vi "Folder Hierarchy Verifier.vi"() -> ()   [LabVIEW 2023]
doc: "Displays a window to view the expected folder hierarchy on disk and and compare it to the actual folder hierarchy."
uses:
  CTLs/Folder Verifier State Data.ctl
  <userlib>/_MGI/Application Control/MGI Gray if/MGI Gray if False.vi
  SubVIs/FaKI State Machine/FaKI State Machine.lvlib
panel:
  in  "Flat Constructors?":bool
  in  "Project Hierarchy":string(tree)
  in  "Analyze Project":bool
  in  "Exit":bool
  in  "Project File":path
  # "A non-container project item will be red if expected path does not match actual path. A container project item will be red if none of the containing expected paths match actual paths, purple if some match and some don't match, and dark red if non-container items directly below it do not share a common directory"
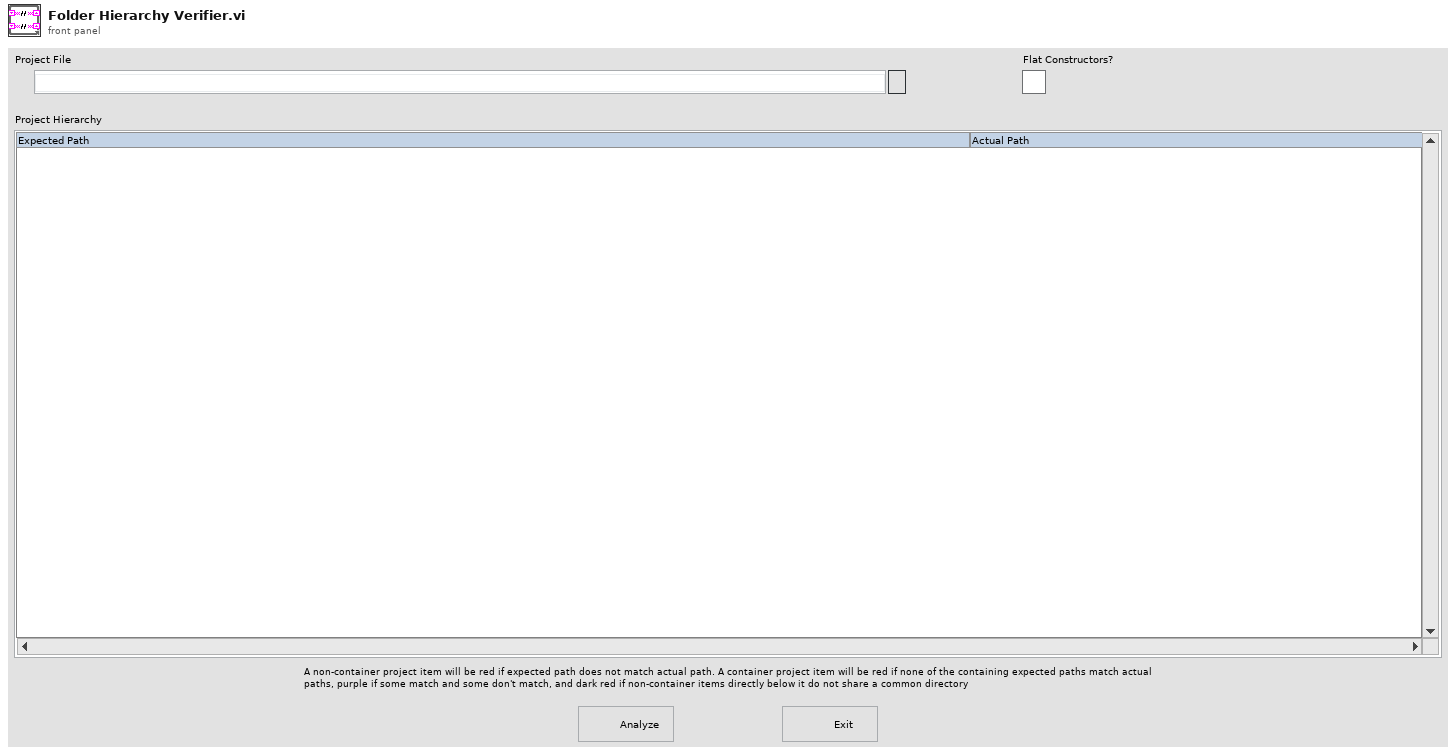
[diagram p1: front panel]
types:
  T1 = typedef "Folder Verifier State Data.ctl" = cluster{"Core":cluster{"Current VI Reference":refnum<vi>, "Close Panel on Exit?":bool}, "Tree Refnum":refnum<vi>, "Project":path, "Expected Paths":path[], "Actual Paths":path[]}
  T2 = enum32{"Invalid", "Standard", "Closed", "Hidden", "Minimized", "Maximized"}
  T3 = enum32{"invalid app kind", "Development System", "Run Time System", "Student Edition", "Embedded LabVIEW", "Evaluation", "Custom"}
  T4 = enum8{"Enabled", "Disabled", "Disabled and Grayed Out"}
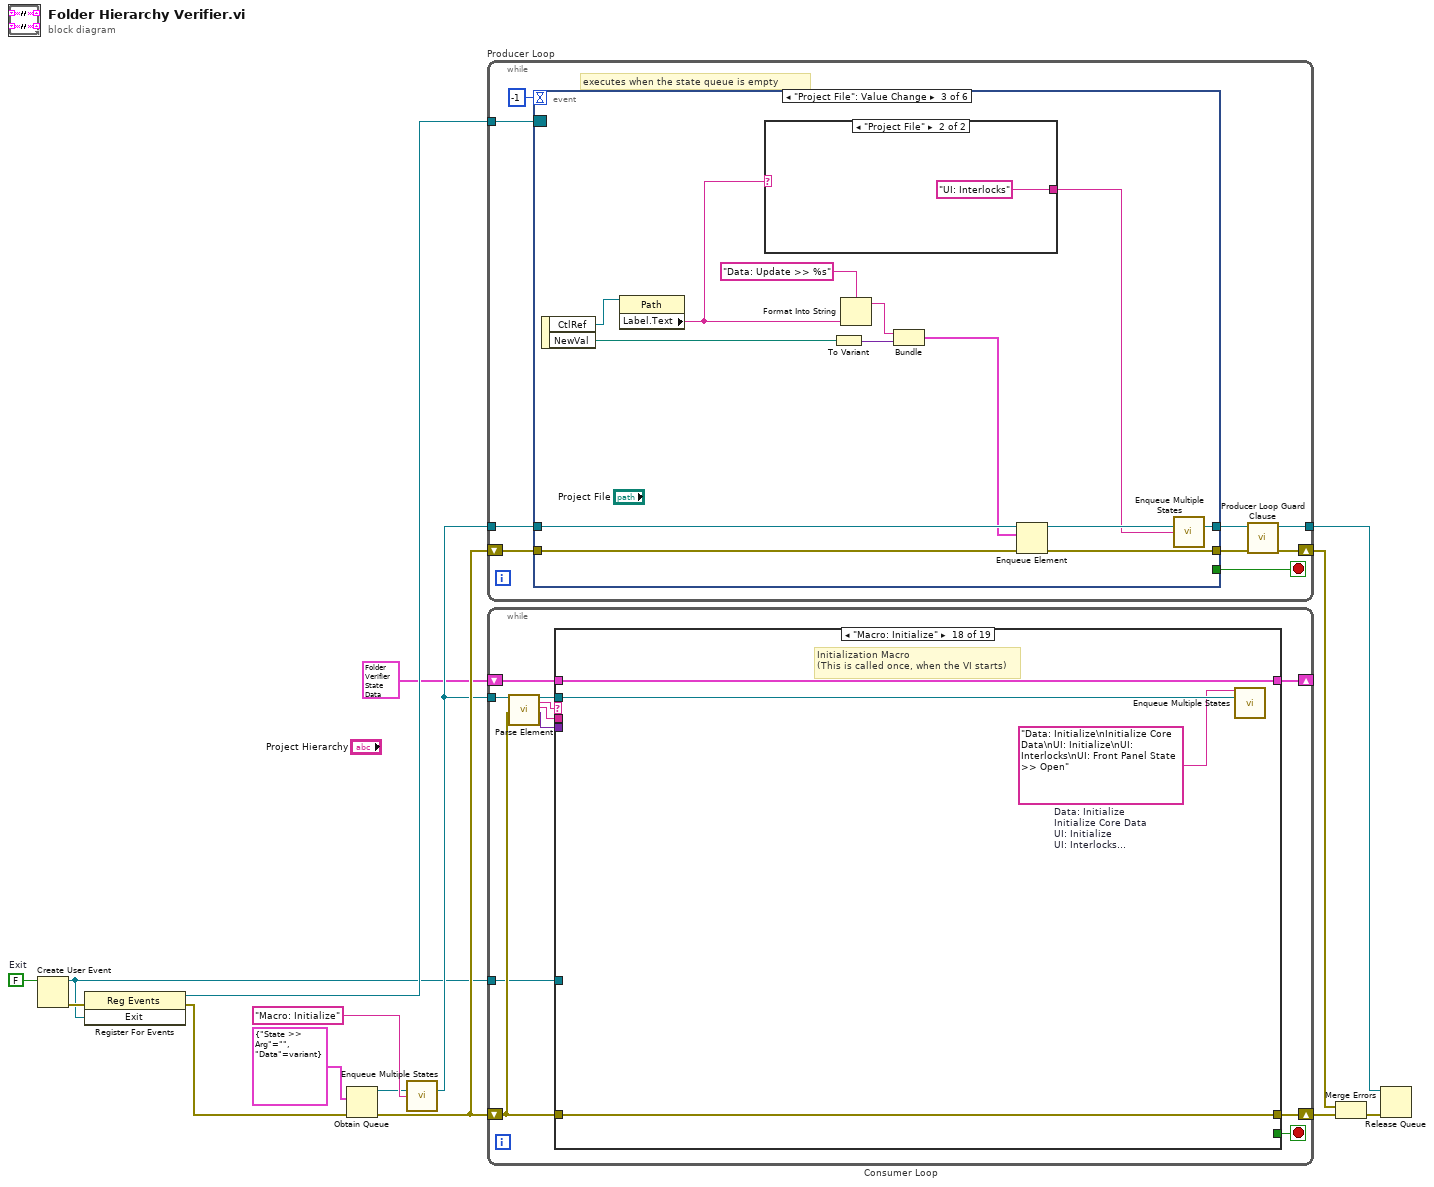
[diagram p0: block diagram]
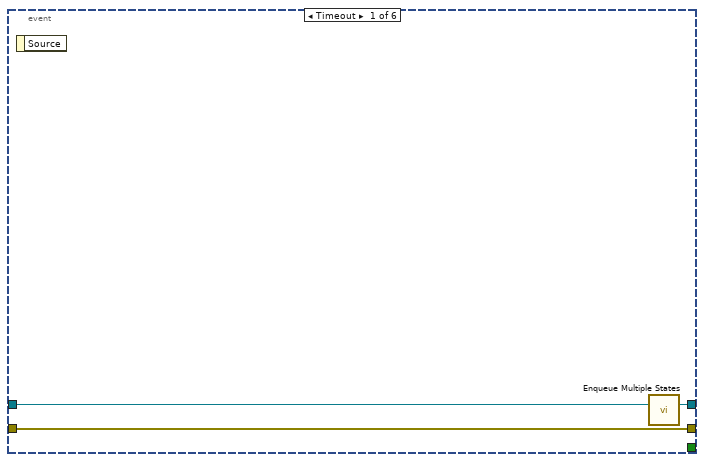
[diagram p2: hidden frame]
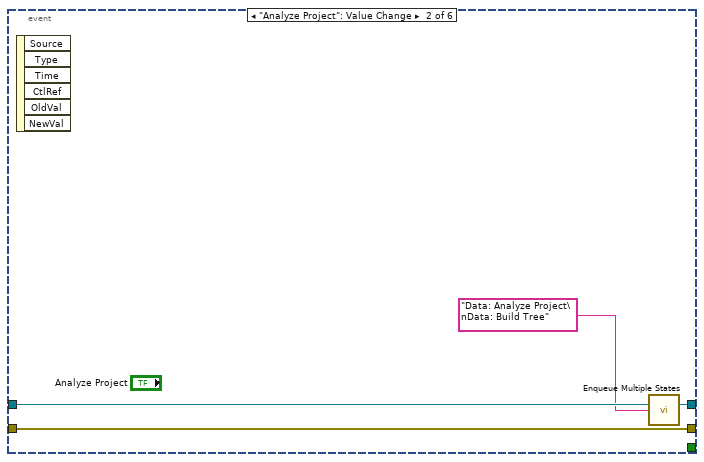
[diagram p3: hidden frame]
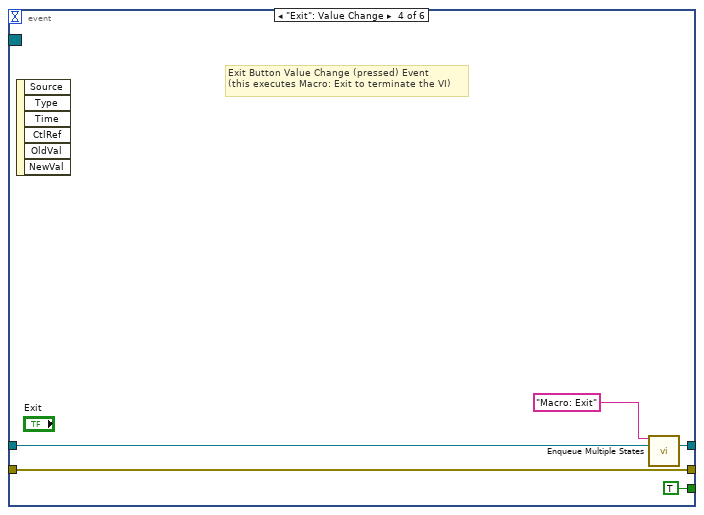
[diagram p5: hidden frame]
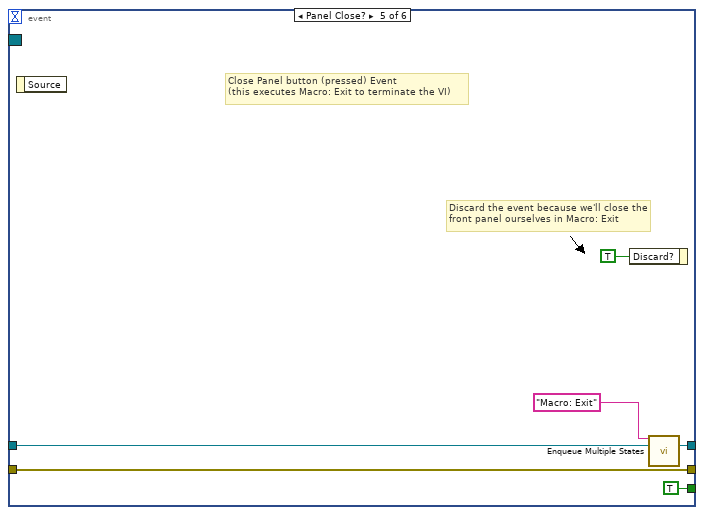
[diagram p6: hidden frame]
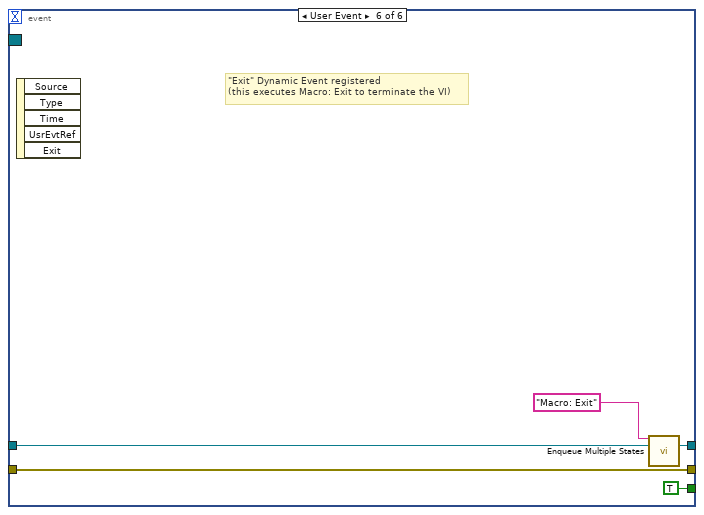
[diagram p7: hidden frame]
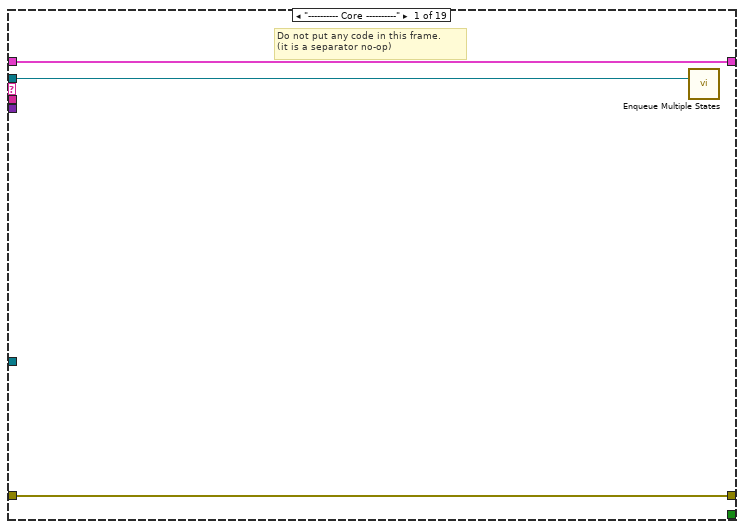
[diagram p8: hidden frame]
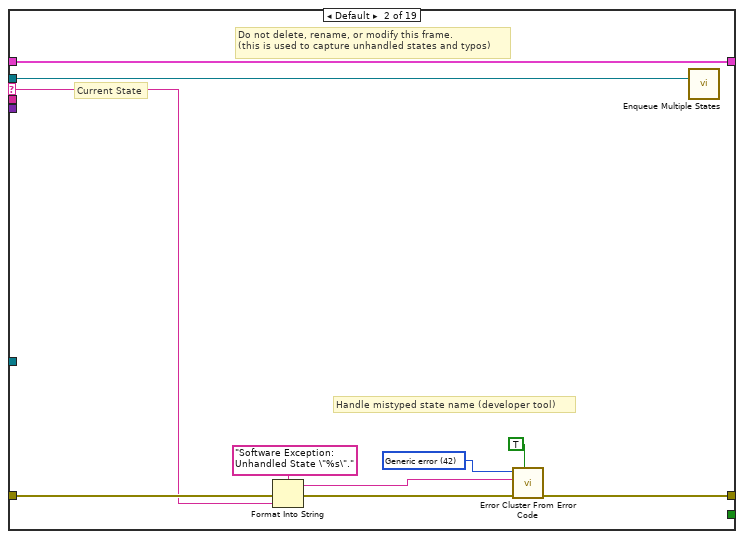
[diagram p9: hidden frame]
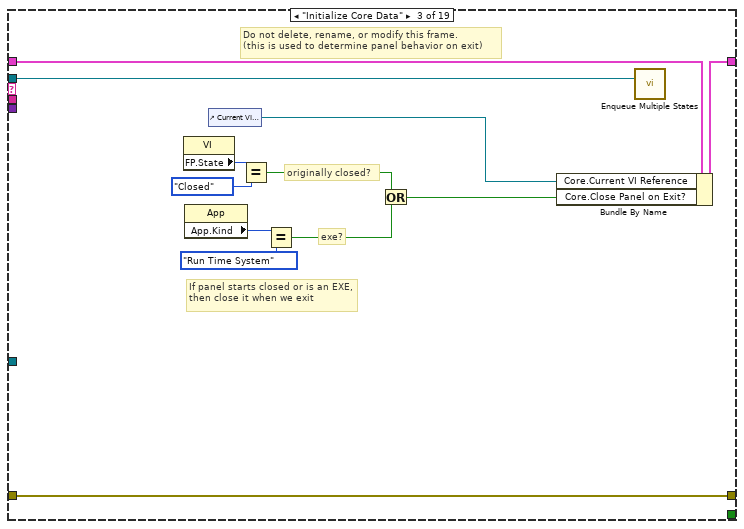
[diagram p10: hidden frame]
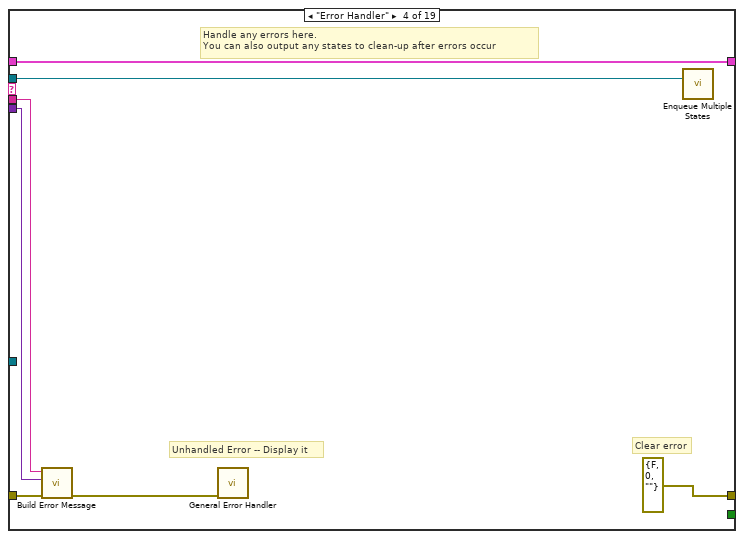
[diagram p11: hidden frame]
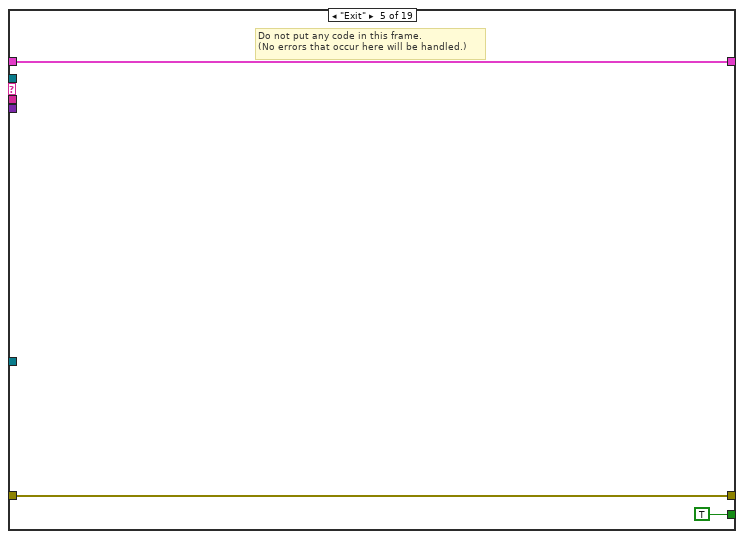
[diagram p12: hidden frame]
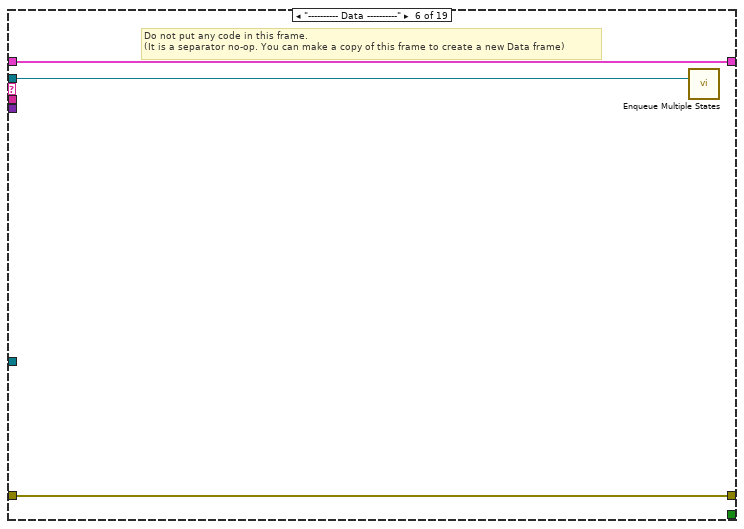
[diagram p13: hidden frame]
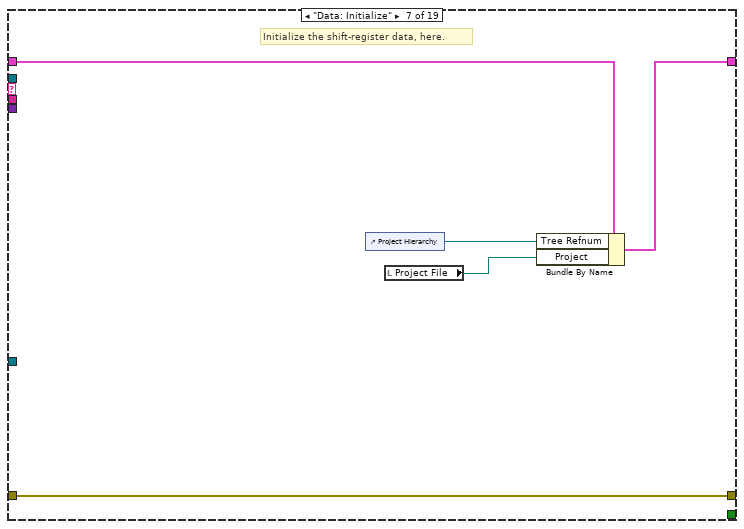
[diagram p14: hidden frame]
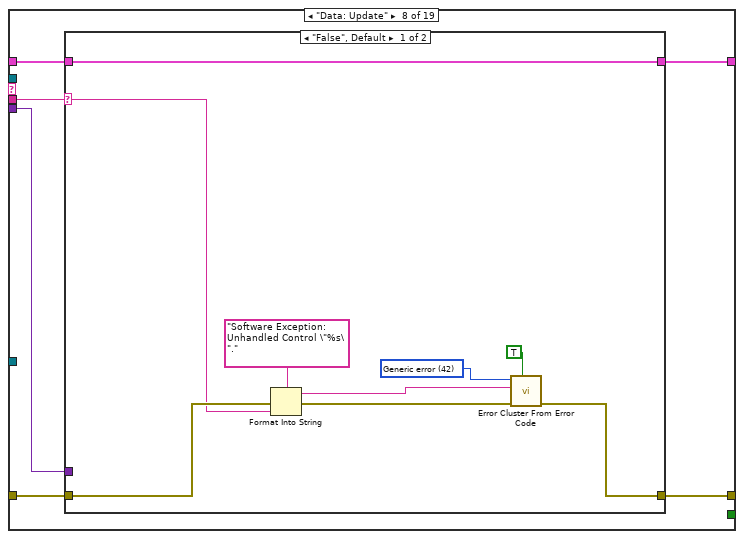
[diagram p15: hidden frame]
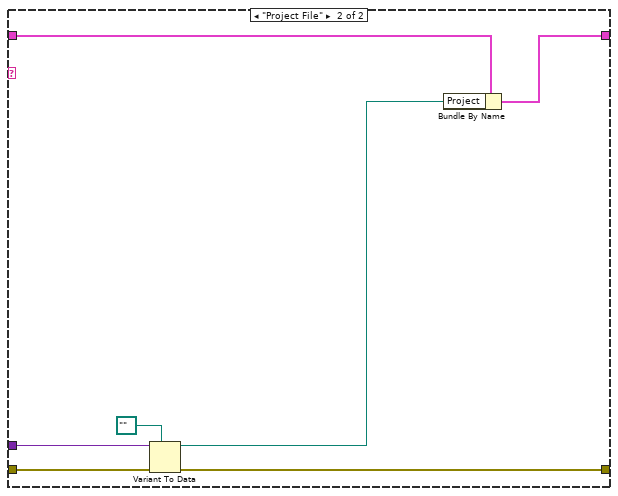
[diagram p16: hidden frame]
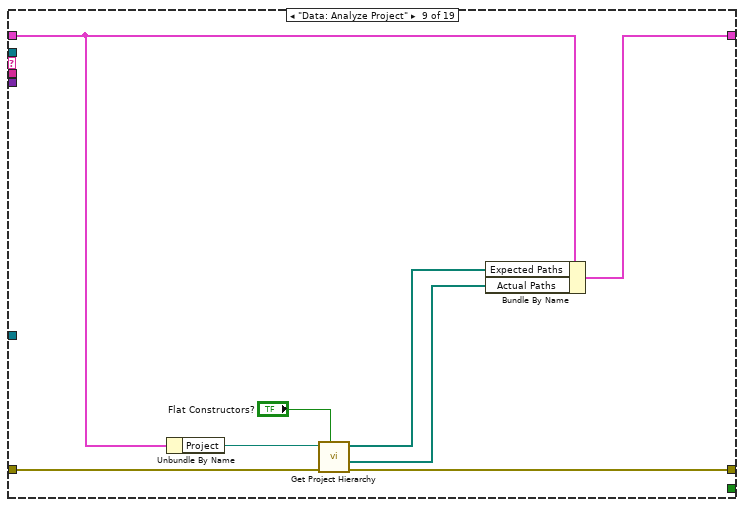
[diagram p17: hidden frame]
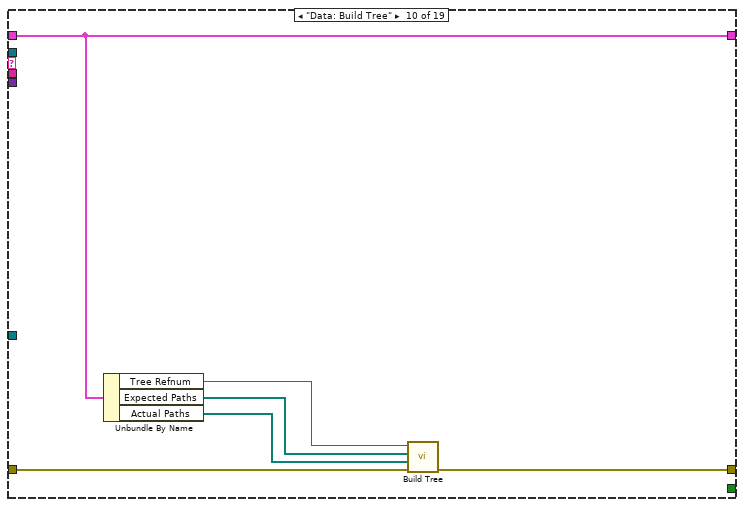
[diagram p18: hidden frame]
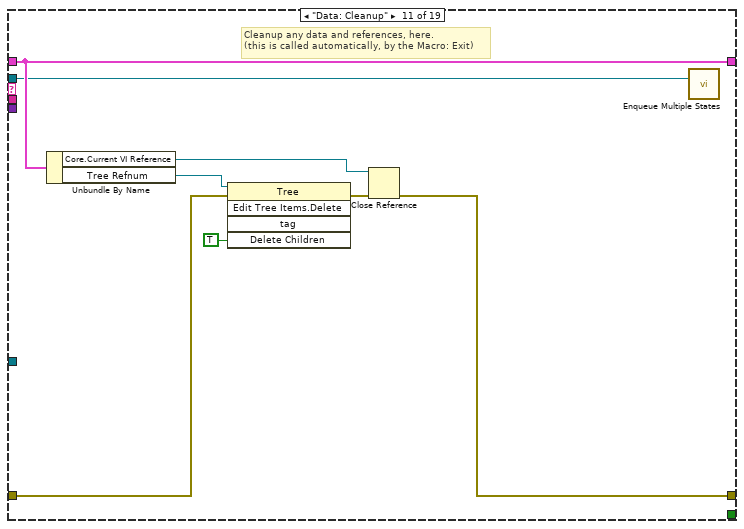
[diagram p19: hidden frame]
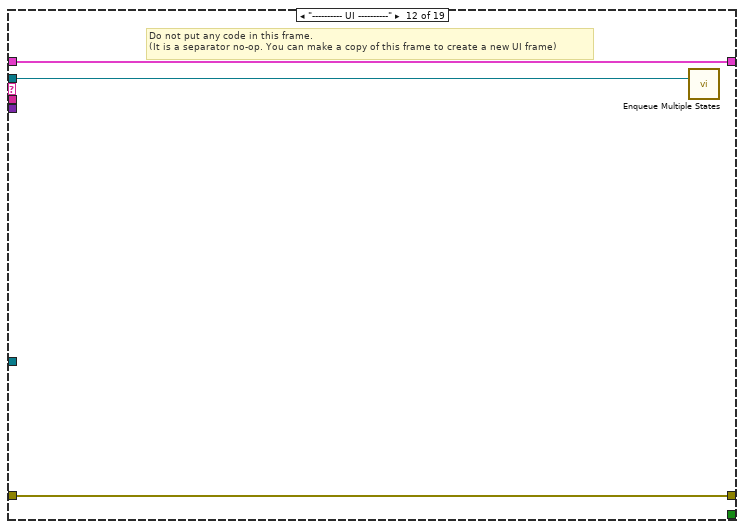
[diagram p20: hidden frame]
diagram:
  w5 = FALSE  # Exit
  n1 = Create User Event(user event datatype=w5) -> (user event=w2:refnum<user-event>, error out=w6:errorcluster)  [unwired: 1 in]
  n2 = register-events(error in=w6, w2) -> (reference out=w3:refnum<event-registration>, error out=w4:errorcluster)  [unwired: 1 in]
  n3 = Obtain Queue(element data type=cluster{"State >> Arg":string, "Data":variant} {"State >> Arg"="", "Data"=variant}, error in (no error)=w4) -> (queue out=w12:refnum<queue>, error out=w15:errorcluster)  [unwired: 3 in, 1 out]
  n4 = call "Enqueue Multiple States.vi"("queue in"=w12, "State(s) at Back"="Macro: Initialize") -> ("queue out"=w11:refnum<queue>)  [unwired: 13 in]
  n5 = while "Producer Loop" {
    shift-right: [w19] -> w9
    shift-left: w15 -> [w24]
    tunnel: w3 -> [w16]
    tunnel: w11 -> [w22]
    tunnel: [w17] -> w7
    stop <- w21 stop-if-true
    # "executes when the state queue is empty"
    n6 = event shown="[2] \"Project File\": Value Change" {
      selector: w16 -> [_ _ _ _ _ _]
      dyn-events: _ -> [_ _ _ _ _ _]
      timeout: -1 ("Timeout") -> [_ _ _ _ _ _]
      tunnel: [w25 w29 w42 w50 w56 w61] -> w20
      tunnel: w24 -> [w25 w29 w43 w50 w56 w61]
      tunnel: w22 -> [w26 w30 w41 w49 w53 w59]
      tunnel: [w27 w31 w44 w47 w52 w58] -> w18
      tunnel: [_ _ _ TRUE TRUE TRUE] -> w21
      event Timeout {
        n7 = event-data() -> ()  [unwired: 1 in, 1 out]
        n8 = call "Enqueue Multiple States.vi"("queue in"=w26) -> ("queue out"=w27:refnum<queue>)  [unwired: 14 in]
      }
      event "Analyze Project": Value Change {
        n9 = event-data() -> ()  [unwired: 1 in, 6 out]
        n10 = call "Enqueue Multiple States.vi"("queue in"=w30, "State(s) at Back"="Data: Analyze Project\nData: Build Tree") -> ("queue out"=w31:refnum<queue>)  [unwired: 13 in]
      }
      event "Project File": Value Change {
        n11 = event-data() -> ("CtlRef"=w39:refnum<vi>, "NewVal"=w38:path)  [unwired: 1 in]
        n12 = property class="Path"(reference=w39) -> ("Label.Text"=w34:string)  [unwired: 1 in, 2 out]
        n13 = case shown="\"Project File\"" w34 {
          tunnel: [_ "UI: Interlocks"] -> w32
          frame "False", Default {
          }
          frame "Project File" {
          }
        }
        n14 = To Variant(anything=w38) -> (Variant=w37:variant)
        n15 = Format Into String(format string="Data: Update >> %s", w34) -> (resulting string=w36:string)  [unwired: 2 in, 1 out]
        n16 = Bundle(w36, "Variant"=w37) -> (w33:cluster{string, "Variant":variant})  [unwired: 1 in]
        n17 = Enqueue Element(queue=w41, element=w33, error in (no error)=w43) -> (queue out=w40:refnum<queue>, error out=w42:errorcluster)  [unwired: 1 in, 1 out]
        n18 = call "Enqueue Multiple States.vi"("queue in"=w40, "State(s) at Back"=w32) -> ("queue out"=w44:refnum<queue>)  [unwired: 13 in]
      }
      event "Exit": Value Change {
        # "Exit Button Value Change (pressed) Event\n(this executes Macro: Exit to terminate the VI)"
        n19 = event-data() -> ()  [unwired: 1 in, 6 out]
        n20 = call "Enqueue Multiple States.vi"("State(s) at Front"="Macro: Exit", "queue in"=w49) -> ("queue out"=w47:refnum<queue>)  [unwired: 13 in]
      }
      event Panel Close? {
        # "Discard the event because we'll close the front panel ourselves in Macro: Exit"
        # "Close Panel button (pressed) Event\n(this executes Macro: Exit to terminate the VI)"
        n21 = event-data() -> ()  [unwired: 1 in, 1 out]
        n22 = event-data("Discard?"=TRUE) -> ()  [unwired: 1 in, 1 out]
        n23 = call "Enqueue Multiple States.vi"("State(s) at Front"="Macro: Exit", "queue in"=w53) -> ("queue out"=w52:refnum<queue>)  [unwired: 13 in]
      }
      event User Event {
        # "\"Exit\" Dynamic Event registered\n(this executes Macro: Exit to terminate the VI)"
        n24 = event-data() -> ()  [unwired: 1 in, 5 out]
        n25 = call "Enqueue Multiple States.vi"("State(s) at Front"="Macro: Exit", "queue in"=w59) -> ("queue out"=w58:refnum<queue>)  [unwired: 13 in]
      }
    }
    n26 = call "Producer Loop Guard Clause.vi"("error in (no error)"=w20, "queue in"=w18) -> ("error out"=w19:errorcluster, "queue out"=w17:refnum<queue>)  [unwired: 8 in]
  }
  n27 = while "Consumer Loop" {
    shift-right: [w69] -> _
    shift-left: T1 {"Core"={"Current VI Reference"=refnum, "Close Panel on Exit?"=FALSE}, "Tree Refnum"=refnum, "Project"=path "", "Expected Paths"=[], "Actual Paths"=[]} ("Folder Verifier State Data") -> [w68]
    shift-right: [w72] -> w10
    shift-left: w15 -> [w71]
    tunnel: w11 -> [w67]
    tunnel: w2 -> [w62]
    stop <- w70 stop-if-true
    n28 = call "Parse Element.vi"("queue in"=w67, "error in (no error)"=w71) -> ("queue out"=w66:refnum<queue>, "State"=w65:string, "Arg"=w64:string, "Data"=w63:variant)  [unwired: 14 in]
    n29 = case shown="\"Macro: Initialize\"" w65 {
      selector: w65 -> [_ w77 _ _ _ _ _ _ _ _ _ _ _ _ _ _ _ _ _]
      tunnel: w66 -> [w73 w76 w86 w102 _ w108 _ _ _ _ w156 w160 w163 _ w172 w181 w252 w256 w262]
      tunnel: w64 -> [_ _ _ w98 _ _ _ w119 _ _ _ _ _ _ w173 w182 _ _ _]
      tunnel: w68 -> [w74 w79 w92 w103 w106 w109 w114 w120 w140 w151 w157 w161 w164 w170 w174 w184 w253 w257 w266]
      tunnel: [w75 w84 w97 errorcluster {"status"=FALSE, "code"=0, "source"=""} ("error out") w107 w110 w115 w117 w144 w146 w159 w162 w165 w171 w175 w185 w254 w258 w267] -> w72
      tunnel: w71 -> [w75 w83 w97 w101 w107 w110 w115 w121 w145 w147 w153 w162 w165 w171 w176 w186 w254 w258 w267]
      tunnel: [_ _ _ _ TRUE _ _ _ _ _ _ _ _ _ _ _ _ _ _] -> w70
      tunnel: [w74 w79 w96 w103 w106 w109 w113 w116 w143 w151 w157 w161 w164 w170 w174 w184 w253 w257 w266] -> w69
      tunnel: w63 -> [_ _ _ w99 _ _ _ w118 _ _ _ _ _ _ _ _ _ _ _]
      tunnel: w62 -> [_ _ _ _ _ _ _ _ _ _ _ _ _ _ _ _ _ _ _]
      frame "---------- Core ----------" {
        # "Do not put any code in this frame.\n(it is a separator no-op)"
        n30 = call "Enqueue Multiple States.vi"("queue in"=w73) -> ()  [unwired: 14 in, 1 out]
      }
      frame Default {
        w81 = 42 items=["No error", "Argument error", "Memory is full", "Out of zone", "End of file", "File already open", "Generic file I/O error", "File not found", "File permission error", "Disk is full", "Duplicate path", "Too many files open", "System feature not enabled", "Resource file not found", "Cannot add resource", "Resource not found", "Image not found", "Image memory error", "Pen does not exist", "Config type invalid", "Config token not found", "Config parse error", "Config memory error", "Bad external code format", "Bad external code offset", "External code not present", "Null window", "Destroy window error", "Null menu", "Print aborted", "Bad print record", "Print driver error", "Windows error during printing", "Memory error during printing", "Print dialog error", "Generic print error", "Invalid device refnum", "Device not found", "Device parameter error", "Device unit error", "Cannot open device", "Device call aborted", "Generic error", "Cancelled by user", "Object ID too low", "Object ID too high", "Object not in heap", "Unknown heap", "Unknown object (invalid DefProc)", "Unknown object (DefProc not in table)", "Message out of range", "Invalid (null) method", "Unknown message", "Manager call not supported", "Bad address", "Network operation in progress", "Network operation timed out", "Connection is busy", "Network attribute not supported", "Network error", "Address in use", "System out of memory", "Connection aborted", "Connection refused", "Not connected", "Already connected", "Connection closed", "Initialization error (interapplication manager)", "Bad occurrence", "Wait on unbound occurrence handler", "Occurrence queue overflow", "Datalog type conflict", "Unused", "Unrecognized type (interapplication manager)", "Memory corrupt", "Failed to make temporary DLL", "Old CIN version", "Drag socket not found", "Failed to load drop-object", "Failed to register OLE object", "Failed to release OLE object", "Format specifier type mismatch", "Unknown format specifier", "Too few format specifiers", "Too many format specifiers", "Scan failed", "Newer CIN version", "Error converting to variant", "Runtime menu error", "Password tampered", "Variant attribute not found", "Incompatible variant data type", "Event data is not available", "Event Store is not present", "Occurrence is not found", "Event Queue is not created", "Event info is not available", "Refnum passed is NULL", "Error retrieving Class GUID", "Error retrieving CoClass GUID", "Error retrieving TypeLib GUID.", "Bad built application magic bytes.", "Specific driver is different from the specific driver associated with the Logical Name.", "There is no session opened to the class driver.", "Max Error", "MAX - Error with config objects", "MAX - Error loading configuration", "MAX - Group not supported"]
        # "Current State"
        # "Do not delete, rename, or modify this frame.\n(this is used to capture unhandled states and typos)"
        # "Handle mistyped state name (developer tool)"
        n31 = Format Into String(format string="Software Exception: Unhandled State \"%s\"." ("message"), error in=w83, w77) -> (resulting string=w80:string, error out=w85:errorcluster)  [unwired: 1 in]
        n32 = call <vilib>:"Error Cluster From Error Code.vi"("show call chain? (False)"=TRUE, "error in (no error)"=w85, "error message (\"\")"=w80, "error code (0)"=w81) -> ("error out"=w84:errorcluster)  [unwired: 5 in]
        n33 = call "Enqueue Multiple States.vi"("queue in"=w76) -> ()  [unwired: 14 in, 1 out]
      }
      frame "Initialize Core Data" {
        # "Do not delete, rename, or modify this frame.\n(this is used to determine panel behavior on exit)"
        # "originally closed?"
        # "exe?"
        # "If panel starts closed or is an EXE, then close it when we exit"
        n34 = property class="VI"() -> ("FP.State"=w89:T2)  [unwired: 2 in, 2 out]
        n35 = property class="App"() -> ("App.Kind"=w95:T3)  [unwired: 2 in, 2 out]
        n36 = control-ref of="Current VI Reference"() -> (w90:refnum<vi>)
        n37 = Equal?(x=w89, y=T2."Closed" ("Front Panel Window:State")) -> (x = y?=w87:bool)
        n38 = Equal?(x=w95, y=T3."Run Time System" ("Application:Kind")) -> (x = y?=w93:bool)
        n39 = Or(x=w87, y=w93) -> (x .or. y?=w91:bool)
        n40 = Bundle By Name(cluster=w92, "Core.Current VI Reference"=w90, "Core.Close Panel on Exit?"=w91) -> (w96:T1)
        n41 = call "Enqueue Multiple States.vi"("queue in"=w86) -> ()  [unwired: 14 in, 1 out]
      }
      frame "Error Handler" {
        # "Unhandled Error -- Display it"
        # "Handle any errors here.\nYou can also output any states to clean-up after errors occur"
        # "Clear error"
        n42 = call "Build Error Message.vi"("error in (no error)"=w101, "Data"=w99, "Arg"=w98) -> ("error out"=w100:errorcluster)  [unwired: 8 in]
        n43 = call <vilib>:"General Error Handler.vi"("error in (no error)"=w100) -> ()  [unwired: 10 in, 5 out]
        n44 = call "Enqueue Multiple States.vi"("queue in"=w102) -> ()  [unwired: 14 in, 1 out]
      }
      frame "Exit" {
        # "Do not put any code in this frame.\n(No errors that occur here will be handled.)"
      }
      frame "---------- Data ----------" {
        # "Do not put any code in this frame.\n(It is a separator no-op. You can make a copy of this frame to create a new Data frame)"
        n45 = call "Enqueue Multiple States.vi"("queue in"=w108) -> ()  [unwired: 14 in, 1 out]
      }
      frame "Data: Initialize" {
        # "Initialize the shift-register data, here."
        n46 = control-ref of="Project Hierarchy"() -> (w112:refnum<vi>)
        n47 = local read "Project File"() -> (w111:path)
        n48 = Bundle By Name(cluster=w114, "Tree Refnum"=w112, "Project"=w111) -> (w113:T1)
      }
      frame "Data: Update" {
        n49 = case shown="\"False\", Default" w119 {
          selector: w119 -> [w122 _]
          tunnel: w121 -> [w124 w136]
          tunnel: w120 -> [w130 w133]
          tunnel: w118 -> [_ w137]
          tunnel: [w123 w134] -> w117
          tunnel: [w130 w132] -> w116
          frame "False", Default {
            w128 = 42 items=["No error", "Argument error", "Memory is full", "Out of zone", "End of file", "File already open", "Generic file I/O error", "File not found", "File permission error", "Disk is full", "Duplicate path", "Too many files open", "System feature not enabled", "Resource file not found", "Cannot add resource", "Resource not found", "Image not found", "Image memory error", "Pen does not exist", "Config type invalid", "Config token not found", "Config parse error", "Config memory error", "Bad external code format", "Bad external code offset", "External code not present", "Null window", "Destroy window error", "Null menu", "Print aborted", "Bad print record", "Print driver error", "Windows error during printing", "Memory error during printing", "Print dialog error", "Generic print error", "Invalid device refnum", "Device not found", "Device parameter error", "Device unit error", "Cannot open device", "Device call aborted", "Generic error", "Cancelled by user", "Object ID too low", "Object ID too high", "Object not in heap", "Unknown heap", "Unknown object (invalid DefProc)", "Unknown object (DefProc not in table)", "Message out of range", "Invalid (null) method", "Unknown message", "Manager call not supported", "Bad address", "Network operation in progress", "Network operation timed out", "Connection is busy", "Network attribute not supported", "Network error", "Address in use", "System out of memory", "Connection aborted", "Connection refused", "Not connected", "Already connected", "Connection closed", "Initialization error (interapplication manager)", "Bad occurrence", "Wait on unbound occurrence handler", "Occurrence queue overflow", "Datalog type conflict", "Unused", "Unrecognized type (interapplication manager)", "Memory corrupt", "Failed to make temporary DLL", "Old CIN version", "Drag socket not found", "Failed to load drop-object", "Failed to register OLE object", "Failed to release OLE object", "Format specifier type mismatch", "Unknown format specifier", "Too few format specifiers", "Too many format specifiers", "Scan failed", "Newer CIN version", "Error converting to variant", "Runtime menu error", "Password tampered", "Variant attribute not found", "Incompatible variant data type", "Event data is not available", "Event Store is not present", "Occurrence is not found", "Event Queue is not created", "Event info is not available", "Refnum passed is NULL", "Error retrieving Class GUID", "Error retrieving CoClass GUID", "Error retrieving TypeLib GUID.", "Bad built application magic bytes.", "Specific driver is different from the specific driver associated with the Logical Name.", "There is no session opened to the class driver.", "Max Error", "MAX - Error with config objects", "MAX - Error loading configuration", "MAX - Group not supported"]
            n50 = Format Into String(format string="Software Exception: Unhandled Control \"%s\"." ("message"), error in=w124, w122) -> (resulting string=w127:string, error out=w129:errorcluster)  [unwired: 1 in]
            n51 = call <vilib>:"Error Cluster From Error Code.vi"("show call chain? (False)"=TRUE, "error in (no error)"=w129, "error message (\"\")"=w127, "error code (0)"=w128) -> ("error out"=w123:errorcluster)  [unwired: 5 in]
          }
          frame "Project File" {
            n52 = Variant To Data(error in=w136, type=path "", Variant=w137) -> (data=w131:path, error out=w134:errorcluster)
            n53 = Bundle By Name(cluster=w133, "Project"=w131) -> (w132:T1)
          }
        }
      }
      frame "Data: Analyze Project" {
        n54 = Unbundle By Name(w140) -> ("Project"=w139:path)
        n55 = call "Get Project Hierarchy.vi"("Flat Constructors?"="Flat Constructors?", "error in (no error)"=w145, "Project Path"=w139) -> ("error out"=w144:errorcluster, "Actual Locations"=w141:path[], "Expected Locations"=w142:path[])  [unwired: 6 in]
        n56 = Bundle By Name(cluster=w140, "Expected Paths"=w142, "Actual Paths"=w141) -> (w143:T1)
      }
      frame "Data: Build Tree" {
        n57 = Unbundle By Name(w151) -> ("Tree Refnum"=w149:refnum<vi>, "Expected Paths"=w150:path[], "Actual Paths"=w148:path[])
        n58 = call "Build Tree.vi"("error in (no error)"=w147, "Actual Path"=w148, "Expected Path"=w150, "Tree Refnum"=w149) -> ("error out"=w146:errorcluster)  [unwired: 6 in, 1 out]
      }
      frame "Data: Cleanup" {
        # "Cleanup any data and references, here.\n(this is called automatically, by the Macro: Exit)"
        n59 = Unbundle By Name(w157) -> ("Core.Current VI Reference"=w158:refnum<vi>, "Tree Refnum"=w155:refnum<vi>)
        n60 = invoke class="Tree" method="Edit Tree Items.Delete"(reference=w155, error in=w153, "Delete Children"=TRUE ("Delete Children?")) -> (error out=w152:errorcluster)  [unwired: 2 in, 4 out]
        n61 = Close Reference(reference=w158, error in (no error)=w152) -> (error out=w159:errorcluster)
        n62 = call "Enqueue Multiple States.vi"("queue in"=w156) -> ()  [unwired: 14 in, 1 out]
      }
      frame "---------- UI ----------" {
        # "Do not put any code in this frame.\n(It is a separator no-op. You can make a copy of this frame to create a new UI frame)"
        n63 = call "Enqueue Multiple States.vi"("queue in"=w160) -> ()  [unwired: 14 in, 1 out]
      }
      frame "UI: Initialize" {
        # "Initialize the User Interface, here.\n(this is called automatically, by the Macro: Init)"
        n64 = call "Enqueue Multiple States.vi"("queue in"=w163) -> ()  [unwired: 14 in, 1 out]
      }
      frame "UI: Interlocks" {
        n65 = Unbundle By Name(w170) -> ("Project"=w167:path)
        n66 = Empty String/Path?(string/path=w167) -> (empty?=w168:bool)
        n67 = Not(x=w168) -> (.not. x?=w166:bool)
        n68 = call-poly <userlib>:"MGI Gray if.vi"("Boolean"=w166) -> ("Disabled"=w169:T4)
        n69 = property on="Analyze Project" class="Bool"("DisabledEnum"=w169) -> ()  [unwired: 2 in, 2 out]
      }
      frame "UI: Cursor Set" {
        # "Argument"
        # "Set and Unset Cursor Busy.\n(Usage: \"UI: Cursor Set >> Busy|Idle\")"
        n70 = case shown="\"Idle\", Default" w173 {
          tunnel: w176 -> [w178 w180]
          tunnel: [w177 w179] -> w175
          frame "Idle", Default {
            n71 = call <vilib>:"Unset Busy.vi"("error in (no error)"=w178) -> ("error out"=w177:errorcluster)  [unwired: 10 in]
          }
          frame "Busy" {
            n72 = call <vilib>:"Set Busy.vi"("error in (no error)"=w180) -> ("error out"=w179:errorcluster)  [unwired: 9 in, 1 out]
          }
        }
        n73 = call "Enqueue Multiple States.vi"("queue in"=w172) -> ()  [unwired: 14 in, 1 out]
      }
      frame "UI: Front Panel State" {
        # "Argument"
        # "Set Front Panel Open or Closed\n(Usage: \"UI: Front Panel State >> Open|Close\")"
        n74 = Unbundle By Name(w184) -> ("Core.Current VI Reference"=w183:refnum<vi>)
        n75 = case shown="\"Open\", \"Standard\", Default" w182 {
          tunnel: w186 -> [w193 w207 w219 w232 w245]
          tunnel: [w194 w208 w220 w233 w246] -> w185
          tunnel: w183 -> [w191 w205 w217 w230 w243]
          frame "Open", "Standard", Default {
            w187 = T2."Standard" ("State")
            n76 = property class="VI"(reference=w191, error in=w193) -> (reference out=w190:refnum<vi>, error out=w192:errorcluster, "FP.State"=w189:T2)
            n77 = Not Equal?(x=w189, y=w187) -> (x != y?=w188:bool)
            n78 = case shown="True" w188 {
              tunnel: [w199 w200] -> w194
              tunnel: w192 -> [w198 w200]
              tunnel: w190 -> [w196 _]
              tunnel: w187 -> [w195 _]
              frame True {
                n79 = invoke class="VI" method="FP.Open"(reference=w196, error in=w198, "Activate"=TRUE, "State"=w195) -> (error out=w199:errorcluster)  [unwired: 1 in, 4 out]
              }
              frame False {
              }
            }
          }
          frame "Close", "Closed" {
            n80 = property class="VI"(reference=w205, error in=w207) -> (reference out=w204:refnum<vi>, error out=w206:errorcluster, "FP.State"=w202:T2)
            n81 = Not Equal?(x=w202, y=T2."Closed" ("Front Panel Window:State")) -> (x != y?=w201:bool)
            n82 = case shown="True" w201 {
              tunnel: [w209 w212] -> w208
              tunnel: w206 -> [w209 w211]
              tunnel: w204 -> [_ w210]
              frame False {
              }
              frame True {
                n83 = invoke class="VI" method="FP.Close"(reference=w210, error in=w211) -> (error out=w212:errorcluster)  [unwired: 1 in, 2 out]
              }
            }
          }
          frame "Hidden", "Hide" {
            w213 = T2."Hidden" ("State")
            n84 = property class="VI"(reference=w217, error in=w219) -> (reference out=w216:refnum<vi>, error out=w218:errorcluster, "FP.State"=w215:T2)
            n85 = Not Equal?(x=w215, y=w213) -> (x != y?=w214:bool)
            n86 = case shown="True" w214 {
              tunnel: [w224 w225] -> w220
              tunnel: w218 -> [w223 w225]
              tunnel: w216 -> [w222 _]
              tunnel: w213 -> [w221 _]
              frame True {
                n87 = invoke class="VI" method="FP.Open"(reference=w222, error in=w223, "State"=w221) -> (error out=w224:errorcluster)  [unwired: 2 in, 4 out]
              }
              frame False {
              }
            }
          }
          frame "Minimize", "Minimized" {
            w226 = T2."Minimized" ("State")
            n88 = property class="VI"(reference=w230, error in=w232) -> (reference out=w229:refnum<vi>, error out=w231:errorcluster, "FP.State"=w228:T2)
            n89 = Not Equal?(x=w228, y=w226) -> (x != y?=w227:bool)
            n90 = case shown="True" w227 {
              tunnel: [w237 w238] -> w233
              tunnel: w231 -> [w236 w238]
              tunnel: w229 -> [w235 _]
              tunnel: w226 -> [w234 _]
              frame True {
                n91 = invoke class="VI" method="FP.Open"(reference=w235, error in=w236, "State"=w234) -> (error out=w237:errorcluster)  [unwired: 2 in, 4 out]
              }
              frame False {
              }
            }
          }
          frame "Maximize", "Maximized" {
            w239 = T2."Maximized" ("State")
            n92 = property class="VI"(reference=w243, error in=w245) -> (reference out=w242:refnum<vi>, error out=w244:errorcluster, "FP.State"=w241:T2)
            n93 = Not Equal?(x=w241, y=w239) -> (x != y?=w240:bool)
            n94 = case shown="True" w240 {
              tunnel: [w250 w251] -> w246
              tunnel: w244 -> [w249 w251]
              tunnel: w242 -> [w248 _]
              tunnel: w239 -> [w247 _]
              frame True {
                n95 = invoke class="VI" method="FP.Open"(reference=w248, error in=w249, "State"=w247) -> (error out=w250:errorcluster)  [unwired: 2 in, 4 out]
              }
              frame False {
              }
            }
          }
        }
        n96 = call "Enqueue Multiple States.vi"("queue in"=w181) -> ()  [unwired: 14 in, 1 out]
      }
      frame "---------- Macro ----------" {
        # "Do not put any code in this frame.\n(It is a separator no-op. You can make a copy of this frame to create a new Macro frame)"
        n97 = call "Enqueue Multiple States.vi"("queue in"=w252) -> ()  [unwired: 14 in, 1 out]
      }
      frame "Macro: Initialize" {
        w255 = "Data: Initialize\nInitialize Core Data\nUI: Initialize\nUI: Interlocks\nUI: Front Panel State >> Open"  # Data: Initialize Initialize Core Data UI: Initialize UI: Interlocks UI: Front Panel State >> Open
        # "Initialization Macro\n(This is called once, when the VI starts)"
        n98 = call "Enqueue Multiple States.vi"("State(s) at Front"=w255, "queue in"=w256) -> ()  [unwired: 13 in, 1 out]
      }
      frame "Macro: Exit" {
        # "Exit Macro\n(This is called once, when the VI exits)"
        n99 = Unbundle By Name(w266) -> ("Core.Close Panel on Exit?"=w265:bool)
        n100 = Select(t="UI: Front Panel State >> Close\n", s=w265, f="") -> (s? t:f=w261:string)
        n101 = Concatenate Strings(w261, "Data: Cleanup\nExit") -> (w259:string)
        n102 = call "Enqueue Multiple States.vi"("State(s) at Front"=w259, "queue in"=w262) -> ()  [unwired: 13 in, 1 out]
      }
    }
  }
  n103 = Merge Errors(w9, w10) -> (w8:errorcluster)
  n104 = Release Queue(queue=w7, error in (no error)=w8) -> ()  [unwired: 1 in, 3 out]
